vi "DataPacker_ReadConnectionDestination.vi"(0 "DataPacker in":refnum<class "DataPacker.lvclass">, 11 "error in (no error)":errorcluster) -> (4 "DataPacker out":refnum<class "DataPacker.lvclass">, 6 "MIDAS Addresss":string, 8 "MIDAS Port":u16, 10 "Connection Attempt":u32, 14 "Frontend Status":string, 15 "error out":errorcluster)   [LabVIEW 2018, in "feGEM DataPacker.lvlib" / "DataPacker.lvclass"]
uses:
  DataPacker.lvclass
  DataPacker.lvclass/DataPacker.ctl
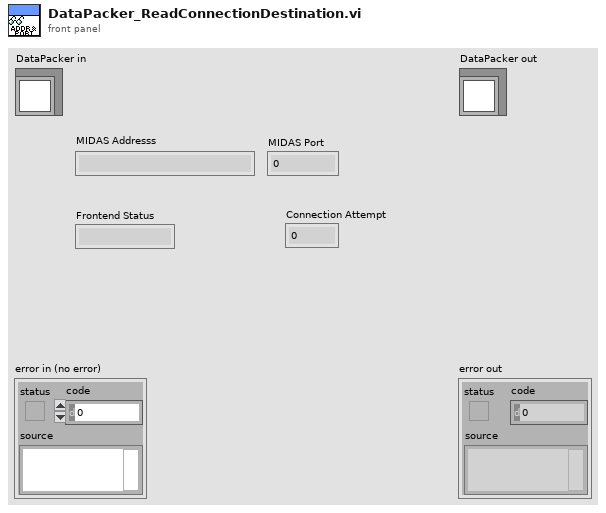
[diagram p1: front panel]
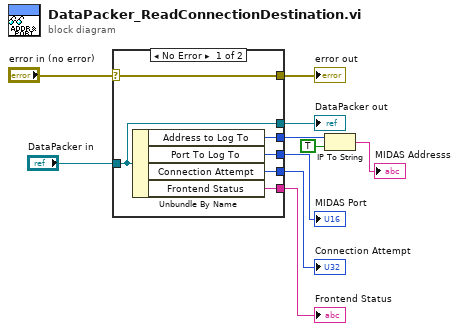
[diagram p0: block diagram]
diagram:
  n1 = case shown="No Error" "error in (no error)" {
    selector: "error in (no error)" -> [w16 w17]
    tunnel: [w16 w17] -> w9
    tunnel: [w15 w18] -> w7
    tunnel: "DataPacker in" -> [w15 w18]
    tunnel: [w14 _] -> w3
    tunnel: [w13 _] -> w6
    tunnel: [w12 _] -> w5
    tunnel: [w11 _] -> w4
    frame No Error {
      n2 = Unbundle By Name(w15) -> ("Address to Log To"=w14:u32, "Port To Log To"=w13:u16, "Connection Attempt"=w12:u32, "Frontend Status"=w11:string)
    }
    frame Error {
    }
  }
  "error out" <- w9
  "DataPacker out" <- w7
  "MIDAS Port" <- w6
  "Connection Attempt" <- w5
  "Frontend Status" <- w4
  n3 = IP To String(1:TRUE ("dot notation? (F)"), 2:w3) -> (0:→"MIDAS Addresss":string)
